vi "_Last Sibling.vi"(8 "error in (no error)":errorcluster, 11 "NodeRef In":refnum<data-value>) -> (0 "error out":errorcluster, 2 "Last Sibling":refnum<data-value>, 3 "NodeRef":refnum<data-value>)   [LabVIEW 2020, in "PicoG-ParserLexer.lvlib" / "Node.lvclass"]
uses:
  Node.lvclass
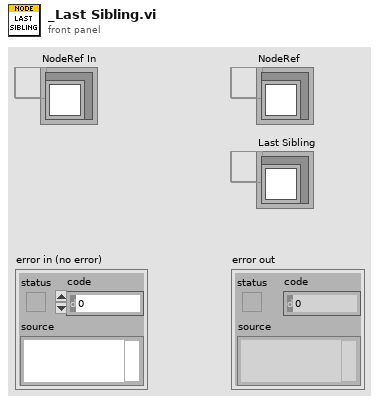
[diagram p1: front panel]
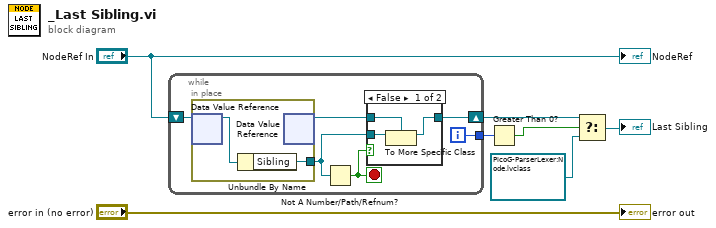
[diagram p0: block diagram]
diagram:
  n1 = while {
    shift-right: [w9] -> w3
    shift-left: "NodeRef In" -> [w13]
    tunnel: [w8] -> w5
    i -> [w8]
    stop <- w12 stop-if-true
    n2 = in-place {
      in-place-border: [w18] -> w11
      n3 = in-place-dvr #1(w13) -> (w19:refnum<class "Node.lvclass">)  [unwired: 1 out]
      n4 = Unbundle By Name(w19) -> ("Sibling"=w18:refnum<data-value>)
      n5 = in-place-dvr #1() -> (w10:refnum<data-value>)  [unwired: 1 in, 1 out]
    }
    n6 = Not A Number/Path/Refnum?(number/path/refnum=w11) -> (NaN/Path/Refnum?=w12:bool)
    n7 = case shown="False" w12 {
      tunnel: w11 -> [w16 _]
      tunnel: w10 -> [w15 w17]
      tunnel: [w14 w17] -> w9
      frame False {
        n8 = To More Specific Class(target class=w15, reference=w16) -> (specific class reference=w14:refnum<data-value>)  [unwired: 1 in, 1 out]
      }
      frame True {
      }
    }
  }
  n9 = Greater Than 0?(x=w5) -> (x > 0?=w2:bool)
  n10 = Select(t=w3, s=w2, f=refnum<data-value> refnum) -> (s? t:f=→"Last Sibling":refnum<data-value>)
  "error out" <- "error in (no error)"
  "NodeRef" <- "NodeRef In"
